vi "Initialize Map.vi"(10 "Column":i32, 11 "Row":i32) -> (3 "map":refnum<data-value>)   [LabVIEW 2015, in "DS Square.lvlib"]
uses:
  DS Square.lvlib
  Map.ctl
  Square Status.ctl
  Square State.ctl
  Center of Mass.ctl
  SubVIs/Read-Only Globals.vi
  SubVIs/Globals (private).vi
  Square/Square.lvclass
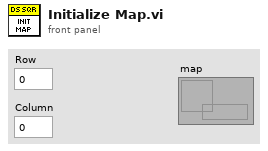
[diagram p1: front panel]
types:
  T1 = typedef "DS Square.lvlib/Center of Mass.ctl" = cluster{"row":dbl, "col":dbl, "mass":dbl}
  T2 = typedef "DS Square.lvlib/Map.ctl" = cluster{"squares":T3[][], "center of mass":T1}
  T3 = typedef "DS Square.lvlib/Square Status.ctl" = cluster{"square state":T4, "probability":dbl, "last update":i32}
  T4 = typedef "DS Square.lvlib/Square State.ctl" = enum16{"Unknown", "Empty", "Occupied - Active", "Occupied - Cool Down", "Attacked", "Enemy", "Enemy Wall"}
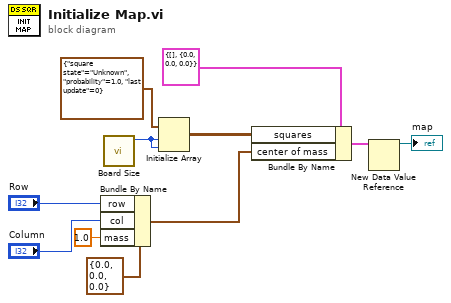
[diagram p0: block diagram]
diagram:
  n1 = Bundle By Name(cluster=T1 {"row"=0.0, "col"=0.0, "mass"=0.0} ("Center of mass"), "row"="Row", "col"="Column", "mass"=1.0) -> (w2:T1)
  n2 = call "Board Size.vi"() -> ("Board Size"=w10:i32)  [unwired: 11 in]
  n3 = Initialize Array(T3 {"square state"=enum."Unknown", "probability"=1.0, "last update"=0} ("square map info"), w10, w10) -> (w8:T3[][])
  n4 = Bundle By Name(cluster=T2 {"squares"=[], "center of mass"={"row"=0.0, "col"=0.0, "mass"=0.0}} ("map"), "squares"=w8, "center of mass"=w2) -> (w7:T2)
  n5 = New Data Value Reference(data value=w7) -> (data value reference=→"map":refnum<data-value>)  [unwired: 1 in, 1 out]
